vi "State Machine.vi"(0 "private data":T1={"GTX2_CHANNEL register map"=refnum, "instruction target"=refnum, "channel measure state"=enum."Uninitialized", "in DFE mode?"=FALSE, "prescale"=0, "rx internal data width"=enum."32 Bit", "active point"={"horizontal offset"=0, "vertical offset"=0}, "ut sign"=enum."Positive", "positive counts"={"sample count"=0, "error count"=0}, "negative counts"={"sample count"=0, "error count"=0}}, 5 "timeout (100 ms)":dbl=0.1, 11 "error in":errorcluster) -> (4 "private data out":T1={"GTX2_CHANNEL register map"=refnum, "instruction target"=refnum, "channel measure state"=enum."Uninitialized", "in DFE mode?"=FALSE, "prescale"=0, "rx internal data width"=enum."32 Bit", "active point"={"horizontal offset"=0, "vertical offset"=0}, "ut sign"=enum."Positive", "positive counts"={"sample count"=0, "error count"=0}, "negative counts"={"sample count"=0, "error count"=0}}, 6 "bit error ratio":dbl, 8 "sample count":u64, 10 "error count":u64, 13 "timed out?":bool, 14 "done?":bool, 15 "error out":errorcluster)   [LabVIEW 2015, in "niHighSpeedSerial Eye Scan Single Point v1 Host.lvclass"]
doc: "Manages the state of the Eye Scan Single Point class and the communication with hardware to obtain measurements on a single point.\n\n<B>Input Parameters</B>\n\n<B>private data</B> is the class private data input into the VI.\n\n<B>private data.GTX2_CHANNEL register map</B> is the GTX2 Channel register map to use.\n\n<B>private data.instruction target</B> is the instruction target to use when communicating with the FPGA.\n\n<B>private data.channel measure state</B> maintains the internal state of the Eye Scan Single Point class.\nenum values: Uninitialized,Initialized,Ready,Request,Wait,Read,Process,Finished\n\n<B>private data.in DFE mode?</B> is true if Eye Scan is configured for DFE Equalization Mode.\n\n<B>private data.prescale</B> controls scaling of the sample count in order to keep the sample count and error count within reasonable precision.\n\n<B>private data.receiver data width</B> is the data width (in bits) of the receiver lane.\nenum values: 16 Bit,20 Bit,32 Bit,40 Bit\n\n<B>private data.active point</B> is the point currently being sampled for errors using Eye Scan.\n\n<B>private data.active point.horizontal offset</B> is the horizontal offset of the active point.\n\n<B>private data.active point.vertical offset</B> is the vertical offset of the active point.\n\n<B>private data.ut sign</B> The untapped threshold sign (positive or negative) currently configured on the point being measured.\nPositive is used when in DFE or LPM Equalization Mode, while Negative is only used in DFE Equalization Mode.\n\n<B>private data.positive counts</B> contains the number of sample and error counts measured using the positive UT Sign.\n\n<B>private data.positive counts.sample count</B> is the positive sample count when using DFE mode, or the entire sample count when using LPM mode.\n\n<B>private data.positive counts.error count</B> is the positive error count when using DFE mode, or the entire error count when using LPM mode.\n\n<B>private data.negative counts</B> contains the number of sample and error counts measured using the negative UT Sign.\n\n<B>private data.negative counts.sample count</B> is the negative sample count when using DFE mode, or unused when using LPM mode.\n\n<B>private data.negative counts.error count</B> is the negative error count when using DFE mode, or unused when using LPM mode.\n\n<B>timeout (100 ms)</B> The amount of time (in seconds) before timing timing out.\nSpecifying '-1' prevents 'timed out' from ever returning true.\n\n<B>error in</B> describes error conditions that occur before this node runs. This input provides standard 'error in' functionality.\n\n<B>Output Parameters</B>\n\n<B>private data out</B> is the class private data output from the VI.\n\n<B>private data out.GTX2_CHANNEL register map</B> is the register map to use which represents the GTX2 Channel.\n\n<B>private data out.instruction target</B> is the instruction target to use when communicating with the FPGA.\n\n<B>private data out.channel measure state</B> maintains the internal state of the Eye Scan Single Point class.\nenum values: Uninitialized,Initialized,Ready,Request,Wait,Read,Process,Finished\n\n<B>private data out.in DFE mode?</B> is true if Eye Scan is configured for DFE Equalization Mode.\n\n<B>private data out.prescale</B> controls scaling of the sample count in order to keep the sample count and error count within reasonable precision.\n\n<B>private data out.receiver data width</B> is the data width (in bits) of the receiver lane.\nenum values: 16 Bit,20 Bit,32 Bit,40 Bit\n\n<B>private data out.active point</B> is the point currently being sampled for errors using Eye Scan.\n\n<B>private data out.active point.horizontal offset</B> is the horizontal offset of the active point.\n\n<B>private data out.active point.vertical offset</B> is the vertical offset of the active point.\n\n<B>private data out.ut sign</B> contains the number of sample and error counts measured using the positive UT Sign.\nenum values: Positive,Negative\n\n<B>private data out.positive counts</B> contains the number of sample and error counts measured using the positive UT Sign.\n\n<B>private data out.positive counts.sample count</B> is the positive sample count when using DFE mode, or the entire sample count when using LPM mode.\n\n<B>private data out.positive counts.error count</B> is the positive error count when using DFE mode, or the entire error count when using LPM mode.\n\n<B>private data out.negative counts</B> contains the number of sample and error counts measured using the negative UT Sign.\n\n<B>private data out.negative counts.sample count</B> is the negative sample count when using DFE mode, or the entire sample count when using LPM mode.\n\n<B>private data out.negative counts.error count</B> is the negative error count when using DFE mode, or the entire error count when using LPM mode.\n\n<B>bit error rate</B> is the calculated statistical bit error rate based on the number of error counts and sample counts received.\n\n<B>sample count</B> is the number of samples that have been measured on this point.\n\n<B>error count</B> is the number of errors that have been measured on this point.\n\n<B>timed out?</B> returns true if at least 'timeout' amount of time has passed.\n\n<B>done?</B> returns true if the Eye Scan algorithm has completed measuring all points.\n\n<B>error out</B> contains error information. This output provides standard 'error out' functionality."
uses:
  <instrlib>/niHighSpeedSerial/Eye Scan/v1/Host/Impl/Single Point/niHighSpeedSerial Eye Scan Single Point v1 Host.lvclass
  <instrlib>/niHighSpeedSerial/Eye Scan/v1/Host/Impl/Single Point/Private/Private Data.ctl
  <instrlib>/niHighSpeedSerial/Register Maps/Xilinx/v1/Host/GTX2_CHANNEL v1 Host.llb/GTX2_CHANNEL Register Map.lvclass
  <instrlib>/_niInstr/Instruction Framework/v1/Host/Instruction Target/niInstr Instruction Target v1 Host.lvclass
  <instrlib>/niHighSpeedSerial/Eye Scan/v1/Host/Impl/Single Point/Private/Channel Measure State.ctl
  <instrlib>/niHighSpeedSerial/Eye Scan/v1/Host/Common/Public/Data Width.ctl
  <instrlib>/niHighSpeedSerial/Eye Scan/v1/Host/Common/Public/Point Offsets.ctl
  <instrlib>/niHighSpeedSerial/Register Maps/Xilinx/v1/Host/GTX2_CHANNEL v1 Host.llb/ESVertOffsetSign.ctl
  <instrlib>/niHighSpeedSerial/Eye Scan/v1/Host/Impl/Single Point/Private/Counts.ctl
  <instrlib>/niHighSpeedSerial/Register Maps/Xilinx/v1/Host/GTX2_CHANNEL v1 Host.llb/GTX2_CHANNEL v1 Host.lvlib
  <instrlib>/niHighSpeedSerial/Eye Scan/v1/Host/Common/niHighSpeedSerial Eye Scan Common v1 Host.lvlib
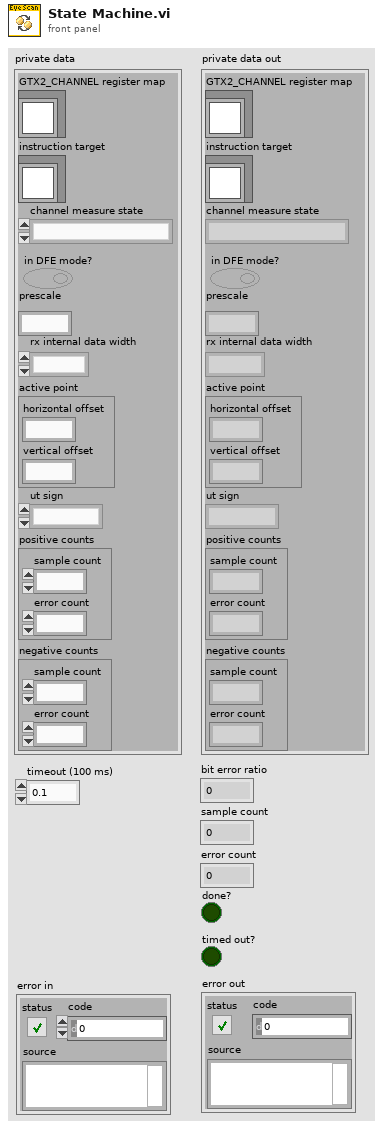
[diagram p1: front panel]
types:
  T1 = typedef "niHighSpeedSerial Eye Scan Single Point v1 Host.lvclass/Private Data.ctl" = cluster{"GTX2_CHANNEL register map":refnum<class "GTX2_CHANNEL Register Map.lvclass">, "instruction target":refnum<class "niInstr Instruction Target v1 Host.lvclass">, "channel measure state":T2, "in DFE mode?":bool, "prescale":u8, "rx internal data width":T3, "active point":T4, "ut sign":T5, "positive counts":T6, "negative counts":T6}
  T2 = typedef "niHighSpeedSerial Eye Scan Single Point v1 Host.lvclass/Channel Measure State.ctl" = enum16{"Uninitialized", "Initialized", "Ready", "Request", "Wait", "Read", "Process", "Finished"}
  T3 = typedef "niHighSpeedSerial Eye Scan Common v1 Host.lvlib/Data Width.ctl" = enum16{"16 Bit", "20 Bit", "32 Bit", "40 Bit"}
  T4 = typedef "niHighSpeedSerial Eye Scan Common v1 Host.lvlib/Point Offsets.ctl" = cluster{"horizontal offset":i16, "vertical offset":i8}
  T5 = typedef "GTX2_CHANNEL v1 Host.lvlib/ESVertOffsetSign.ctl" = enum8{"Positive", "Negative"}
  T6 = typedef "niHighSpeedSerial Eye Scan Single Point v1 Host.lvclass/Counts.ctl" = cluster{"sample count":u64, "error count":u16}
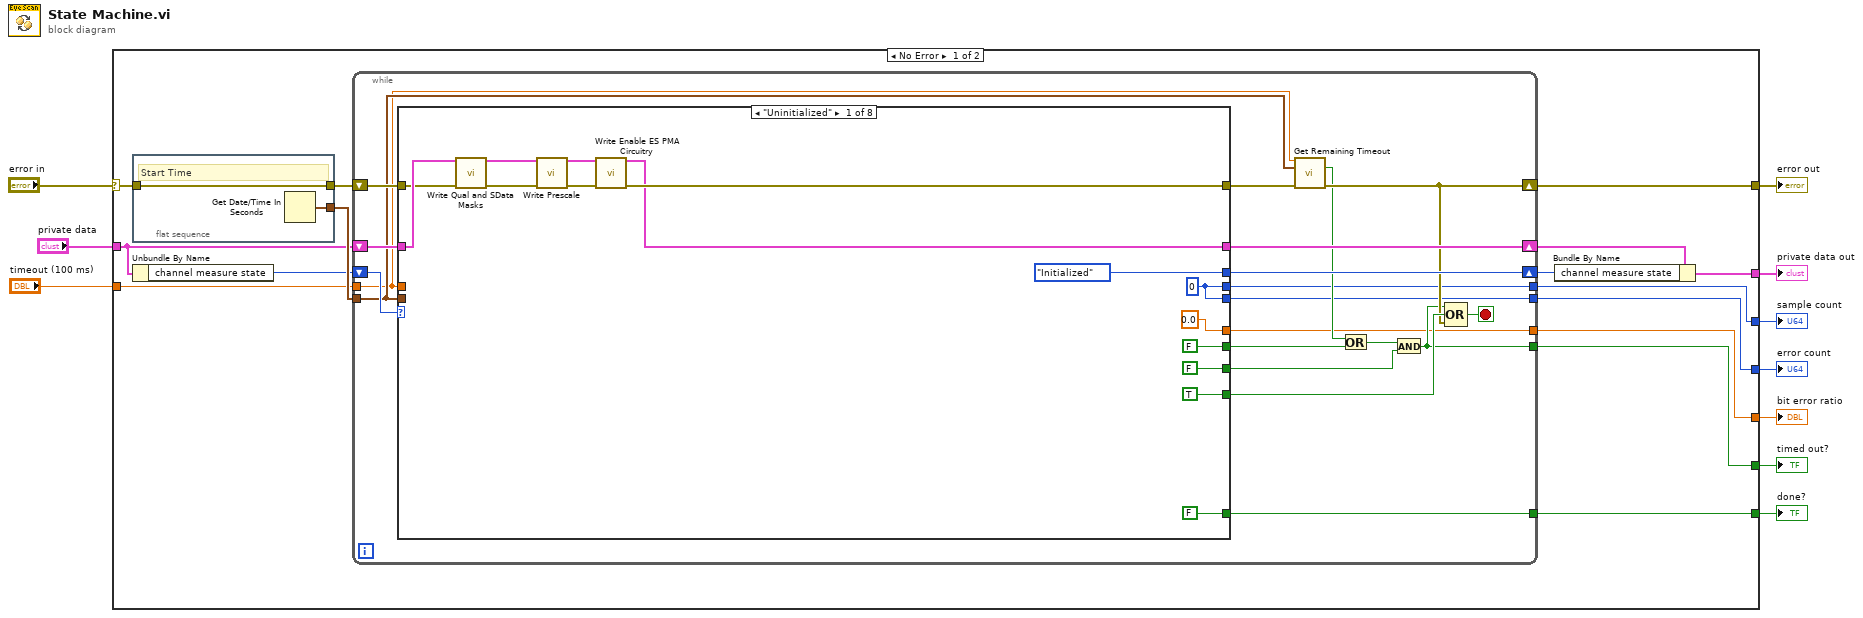
[diagram p0: block diagram]
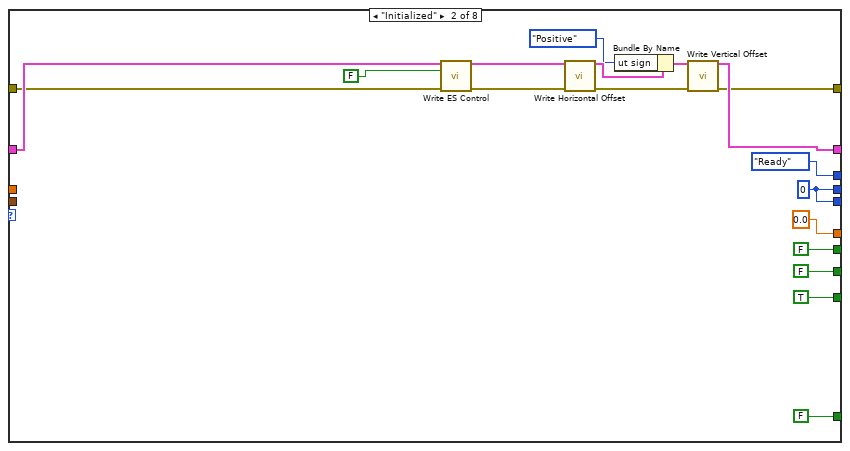
[diagram p2: hidden frame]
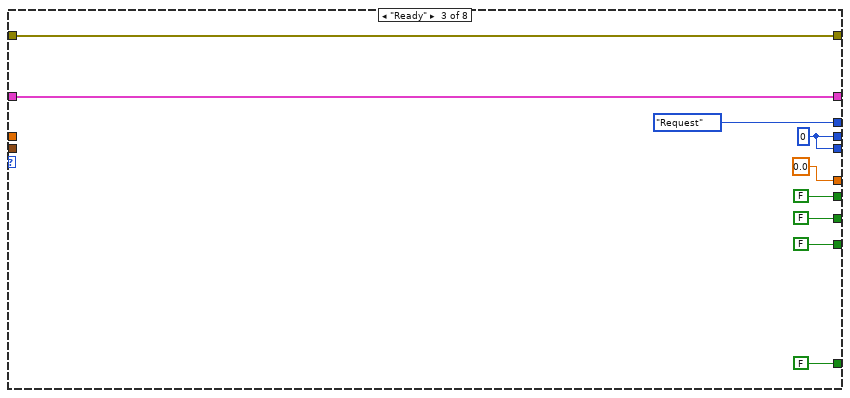
[diagram p3: hidden frame]
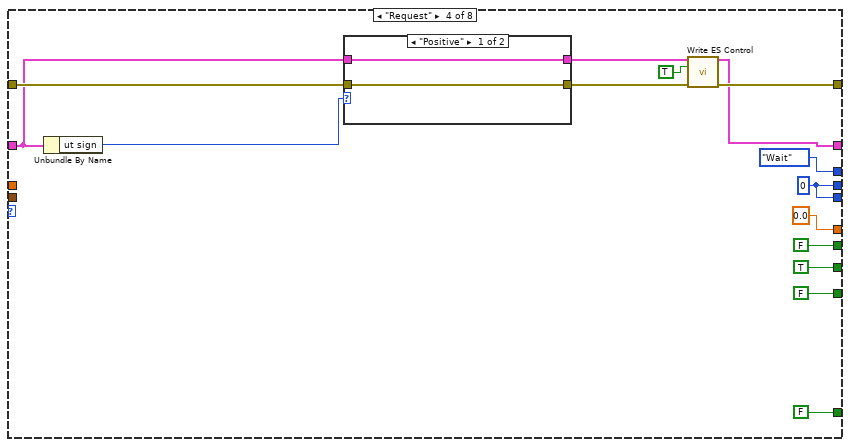
[diagram p4: hidden frame]
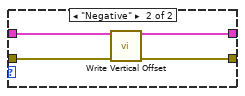
[diagram p5: hidden frame]
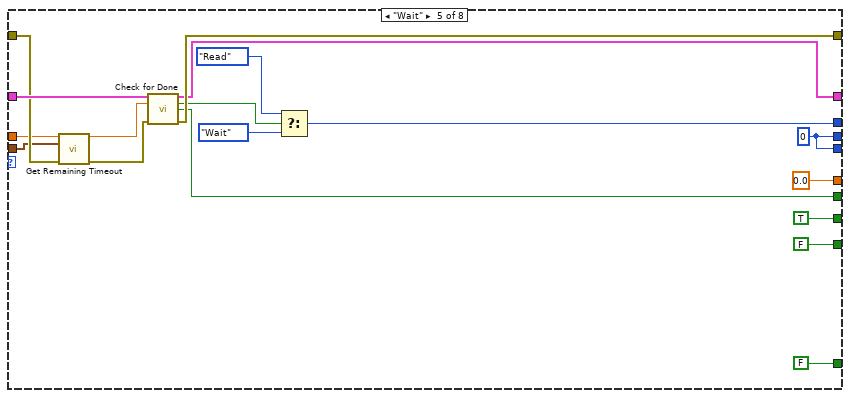
[diagram p6: hidden frame]
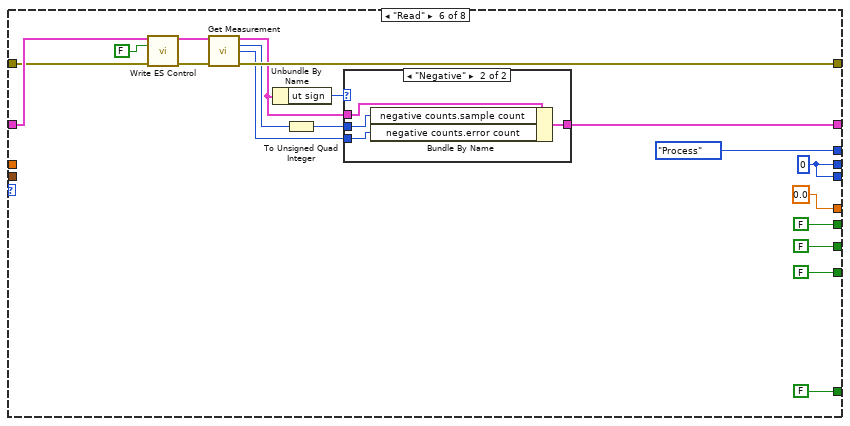
[diagram p7: hidden frame]
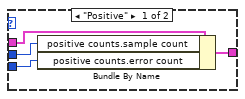
[diagram p8: hidden frame]
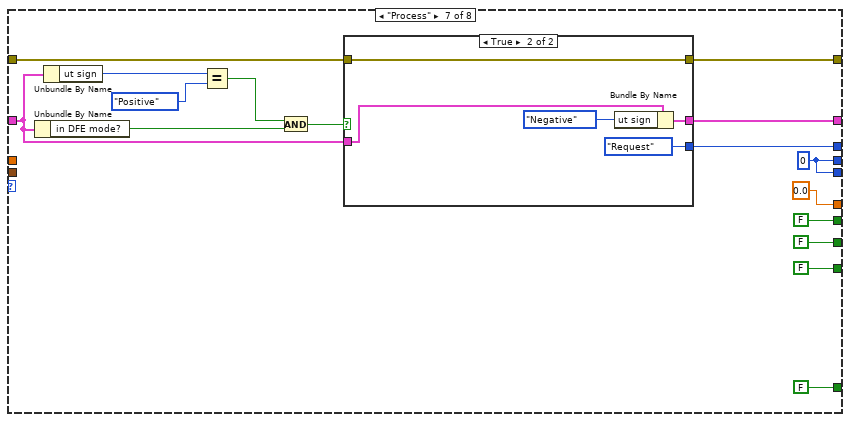
[diagram p9: hidden frame]
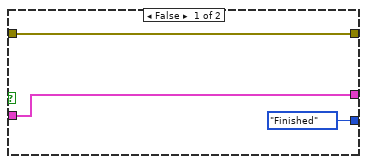
[diagram p10: hidden frame]
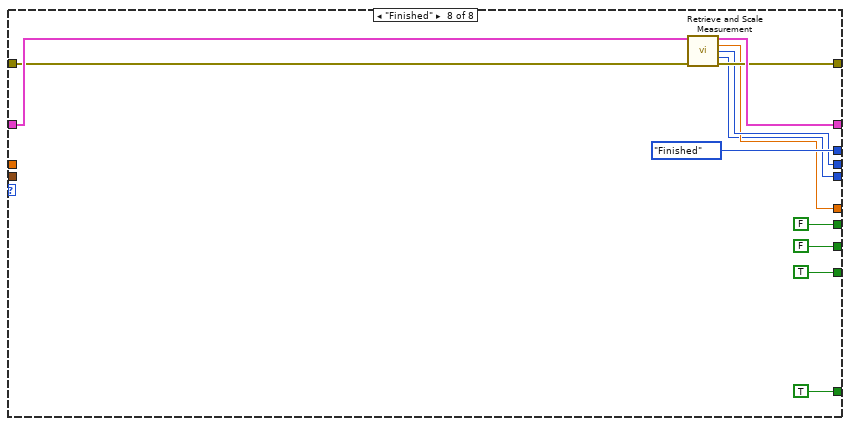
[diagram p11: hidden frame]
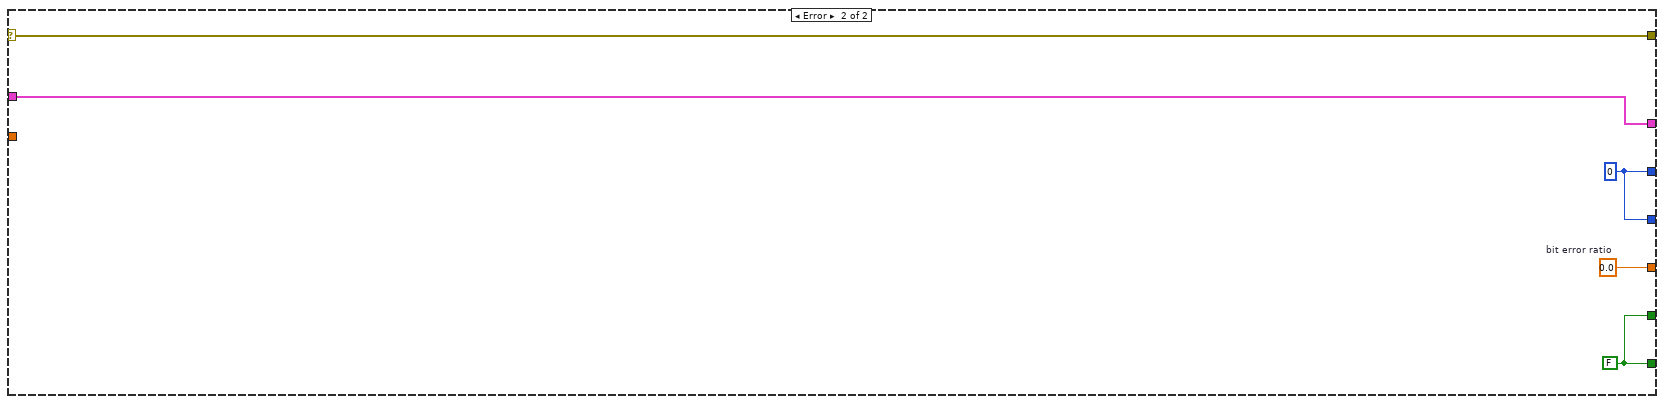
[diagram p12: hidden frame]
diagram:
  n1 = case shown="No Error" "error in" {
    selector: "error in" -> [w24 w196]
    tunnel: [w25 w196] -> w9
    tunnel: "private data" -> [w18 w194]
    tunnel: "timeout (100 ms)" -> [w19 _]
    tunnel: [w21 w195] -> w7
    tunnel: [w20 w195] -> w6
    tunnel: [w14 w194] -> w4
    tunnel: [w13 w193] -> w3
    tunnel: [w12 w192] -> w2
    tunnel: [w11 w193] -> w1
    frame No Error {
      n2 = flat-sequence {
        tunnel: w24 -> [w27]
        tunnel: [w27] -> w22
        tunnel: [w26] -> w23
        frame #0 {
          # "Start Time"
          n3 = Get Date/Time In Seconds() -> (seconds since 1Jan1904=w26:timestamp)
        }
      }
      n4 = Unbundle By Name(w18) -> ("channel measure state"=w17:T2)
      n5 = while {
        tunnel: w19 -> [w39]
        tunnel: w23 -> [w40]
        shift-right: [w35] -> w25
        shift-left: w22 -> [w46]
        tunnel: [w31] -> w21
        tunnel: [w36] -> w20
        shift-right: [w42] -> w15
        shift-left: w17 -> [w43]
        shift-right: [w45] -> w16
        shift-left: w18 -> [w47]
        tunnel: [w30] -> w13
        tunnel: [w29] -> w12
        tunnel: [w28] -> w11
        stop <- w37 stop-if-true
        n6 = case shown="\"Uninitialized\"" w43 {
          tunnel: w47 -> [w53 w73 w88 w96 w126 w147 w160 w188]
          tunnel: w46 -> [w52 w71 w89 w103 w123 w146 w164 w187]
          tunnel: [w55 w79 w88 w97 w125 w138 w165 w186] -> w45
          tunnel: [w59 w78 w89 w98 w128 w143 w163 w185] -> w41
          tunnel: [Channel_Measure_State."Initialized" ("Channel Measure State") Channel_Measure_State."Ready" ("Channel Measure State") Channel_Measure_State."Request" ("Channel Measure State") Channel_Measure_State."Wait" ("Channel Measure State") w115 Channel_Measure_State."Process" ("Channel Measure State") w161 Channel_Measure_State."Finished" ("Channel Measure State")] -> w42
          tunnel: [TRUE TRUE FALSE FALSE FALSE FALSE FALSE TRUE] -> w38
          tunnel: [FALSE FALSE ("Timed out?") FALSE FALSE w124 FALSE ("Timed out?") FALSE ("Timed out?") FALSE ("Timed out?")] -> w44
          tunnel: [FALSE FALSE FALSE FALSE FALSE FALSE FALSE TRUE] -> w36
          tunnel: w39 -> [_ _ _ _ w120 _ _ _]
          tunnel: w40 -> [_ _ _ _ w121 _ _ _]
          tunnel: [FALSE FALSE FALSE TRUE TRUE FALSE FALSE FALSE] -> w32
          tunnel: [w49 w64 w82 w91 w112 w129 w157 w182] -> w30
          tunnel: [0.0 ("bit error ratio") 0.0 ("bit error ratio") 0.0 ("bit error ratio") 0.0 ("bit error ratio") 0.0 ("bit error ratio") 0.0 ("bit error ratio") 0.0 ("bit error ratio") w181] -> w29
          tunnel: [w49 w64 w82 w91 w112 w129 w157 w180] -> w28
          frame "Uninitialized" {
            w49 = u64 0 ("error count")
            n7 = call <instrlib>:"Write Qual and SData Masks.vi"("private data"=w53, "error in"=w52) -> ("private data out"=w61:T1, "error out"=w51:errorcluster)  [unwired: 12 in]
            n8 = call <instrlib>:"Write Prescale.vi"("private data"=w61, "error in"=w51) -> ("private data out"=w60:T1, "error out"=w62:errorcluster)  [unwired: 12 in]
            n9 = call <instrlib>:"Write Enable ES PMA Circuitry.vi"("private data"=w60, "error in"=w62) -> ("private data out"=w55:T1, "error out"=w59:errorcluster)  [unwired: 12 in]
          }
          frame "Initialized" {
            w64 = u64 0 ("sample count")
            n10 = call <instrlib>:"Write ES Control.vi"("private data"=w73, "run?"=FALSE ("Run?"), "error in"=w71) -> ("private data out"=w72:T1, "error out"=w70:errorcluster)  [unwired: 11 in]
            n11 = call <instrlib>:"Write Horizontal Offset.vi"("private data"=w72, "error in"=w70) -> ("private data out"=w69:T1, "error out"=w80:errorcluster)  [unwired: 12 in]
            n12 = Bundle By Name(cluster=w69, "ut sign"=ESVertOffsetSign."Positive" ("ES_VERT_OFFSET_UT_SIGN")) -> (w67:T1)
            n13 = call <instrlib>:"Write Vertical Offset.vi"("private data"=w67, "error in"=w80) -> ("private data out"=w79:T1, "error out"=w78:errorcluster)  [unwired: 12 in]
          }
          frame "Ready" {
            w82 = u64 0 ("sample count")
          }
          frame "Request" {
            w91 = u64 0 ("sample count")
            n14 = Unbundle By Name(w96) -> ("ut sign"=w95:T5)
            n15 = case shown="\"Positive\"" w95 {
              tunnel: w96 -> [w105 w107]
              tunnel: w103 -> [w106 w110]
              tunnel: [w105 w109] -> w100
              tunnel: [w106 w108] -> w99
              frame "Positive" {
              }
              frame "Negative" {
                n16 = call <instrlib>:"Write Vertical Offset.vi"("private data"=w107, "error in"=w110) -> ("private data out"=w109:T1, "error out"=w108:errorcluster)  [unwired: 12 in]
              }
            }
            n17 = call <instrlib>:"Write ES Control.vi"("private data"=w100, "run?"=TRUE ("ES_CONTROL_RUN"), "error in"=w99) -> ("private data out"=w97:T1, "error out"=w98:errorcluster)  [unwired: 11 in]
          }
          frame "Wait" {
            w112 = u64 0 ("sample count")
            n18 = call <instrlib>:"Get Remaining Timeout.vi"("timeout (100 ms)"=w120, "start time"=w121, "error in"=w123) -> ("remaining timeout"=w119:dbl, "error out"=w122:errorcluster)  [unwired: 10 in, 1 out]
            n19 = call <instrlib>:"Check for Done.vi"("private data"=w126, "timeout (100 ms)"=w119, "error in"=w122) -> ("private data out"=w125:T1, "done?"=w118:bool, "timed out?"=w124:bool, "error out"=w128:errorcluster)  [unwired: 8 in, 1 out]
            n20 = Select(t=Channel_Measure_State."Read" ("Channel Measure State"), s=w118, f=Channel_Measure_State."Wait" ("Channel Measure State")) -> (s? t:f=w115:T2)
          }
          frame "Read" {
            w129 = u64 0 ("sample count")
            n21 = call <instrlib>:"Write ES Control.vi"("private data"=w147, "run?"=FALSE ("Run?"), "error in"=w146) -> ("private data out"=w144:T1, "error out"=w145:errorcluster)  [unwired: 11 in]
            n22 = call <instrlib>:"Get Measurement.vi"("private data"=w144, "error in"=w145) -> ("private data out"=w133:T1, "sample count"=w137:u16, "error count"=w136:u16, "error out"=w143:errorcluster)  [unwired: 10 in]
            n23 = Unbundle By Name(w133) -> ("ut sign"=w134:T5)
            n24 = To Unsigned Quad Integer(1:w137) -> (0:w131:u64)
            n25 = case shown="\"Negative\"" w134 {
              tunnel: w133 -> [w151 w155]
              tunnel: [w150 w154] -> w138
              tunnel: w131 -> [w149 w153]
              tunnel: w136 -> [w148 w152]
              frame "Positive" {
                n26 = Bundle By Name(cluster=w151, "positive counts.sample count"=w149, "positive counts.error count"=w148) -> (w150:T1)
              }
              frame "Negative" {
                n27 = Bundle By Name(cluster=w155, "negative counts.sample count"=w153, "negative counts.error count"=w152) -> (w154:T1)
              }
            }
          }
          frame "Process" {
            w157 = u64 0 ("sample count")
            n28 = Unbundle By Name(w160) -> ("in DFE mode?"=w168:bool)
            n29 = Unbundle By Name(w160) -> ("ut sign"=w159:T5)
            n30 = Equal?(x=w159, y=ESVertOffsetSign."Positive") -> (x = y?=w166:bool)
            n31 = And(x=w166, y=w168) -> (x .and. y?=w162:bool)
            n32 = case shown="True" w162 {
              tunnel: w160 -> [w174 w177]
              tunnel: [w174 w175] -> w165
              tunnel: w164 -> [w173 w179]
              tunnel: [w173 w179] -> w163
              tunnel: [Channel_Measure_State."Finished" ("Channel Measure State") Channel_Measure_State."Request" ("Channel Measure State")] -> w161
              frame False {
              }
              frame True {
                n33 = Bundle By Name(cluster=w177, "ut sign"=ESVertOffsetSign."Negative" ("y")) -> (w175:T1)
              }
            }
          }
          frame "Finished" {
            n34 = call <instrlib>:"Retrieve and Scale Measurement.vi"("private data"=w188, "error in"=w187) -> ("private data out"=w186:T1, "bit error ratio"=w181:dbl, "sample count"=w182:u64, "error count"=w180:u64, "error out"=w185:errorcluster)  [unwired: 9 in]
          }
        }
        n35 = call <instrlib>:"Get Remaining Timeout.vi"("timeout (100 ms)"=w39, "start time"=w40, "error in"=w41) -> ("timed out?"=w34:bool, "error out"=w35:errorcluster)  [unwired: 10 in, 1 out]
        n36 = Or(x=w34, y=w44) -> (x .or. y?=w33:bool)
        n37 = And(x=w33, y=w32) -> (x .and. y?=w31:bool)
        n38 = Compound Arithmetic op=OR(w31, w38, w35) -> (w37:bool)
      }
      n39 = Bundle By Name(cluster=w16, "channel measure state"=w15) -> (w14:T1)
    }
    frame Error {
      w192 = 0.0  # bit error ratio
      w193 = u64 0 ("sample count")
      w195 = FALSE ("done")
    }
  }
  "error out" <- w9
  "done?" <- w6
  "timed out?" <- w7
  "private data out" <- w4
  "bit error ratio" <- w2
  "sample count" <- w3
  "error count" <- w1
